vi "Renishaw-XL80_GetDX10Status.vi"(8 "error in (no error)":errorcluster, 11 "Renishaw-XL80_EMU in":refnum<class "Renishaw-XL80_EMU.lvclass">) -> (0 "error out":errorcluster, 2 "DX10Status":i32(ring) items=["DX10_CONNECTED", "DX10_NOT_RESPONDING"], 3 "Renishaw-XL80_EMU out":refnum<class "Renishaw-XL80_EMU.lvclass">)   [LabVIEW 2024, in "Renishaw-XL80_EMU.lvclass"]
doc: "DX10Status property\nThis read only property returns the current status of the DX10. It indicates whether or not the DX10 is responding.\n\nDefinition\nHRESULT\nget_DX10Status(\n [out, retval] DX10_STATUS_CODES* pVal\n);\n\nParameters\npVal\nA variable that will be set one of the DX10_STATUS_CODES.\n\nComments\nThis property will return with an HRESULT of E_FAIL if the client has not previously connected to a DX10 by calling Connect.\n\nThe property will normally return an HRESULT of S_OK. However, it will return E_POINTER if the client supplies a null pointer for pVal.\n\nNote: if there is a XL laser connected to the DX10Adaptor COM interface this property relates to a virtual DX10 and will always return DX10_CONNECTED."
uses:
  Renishaw-XL80_EMU.lvclass
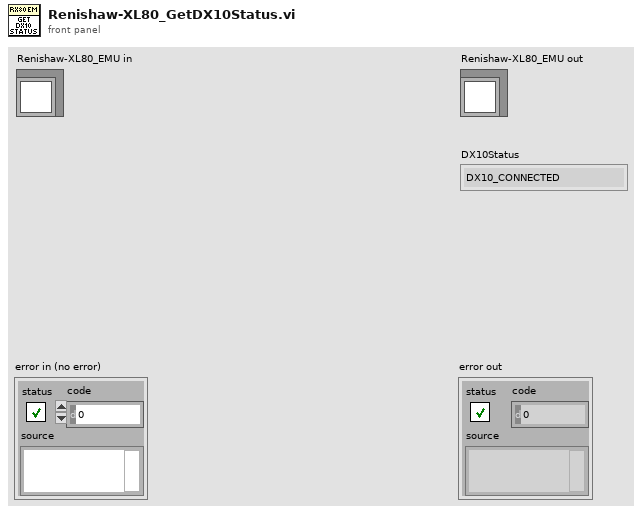
[diagram p1: front panel]
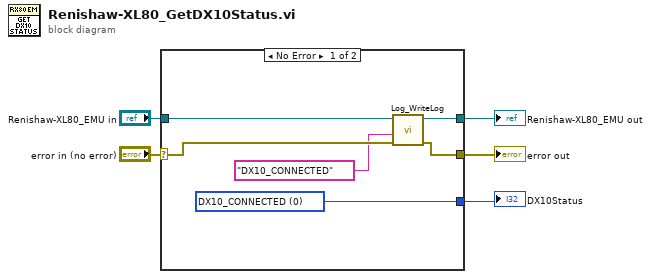
[diagram p0: block diagram]
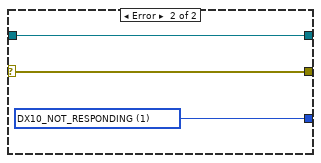
[diagram p2: hidden frame]
diagram:
  n1 = case shown="No Error" "error in (no error)" {
    selector: "error in (no error)" -> [w7 w13]
    tunnel: "Renishaw-XL80_EMU in" -> [w8 w14]
    tunnel: [w10 w14] -> w4
    tunnel: [w9 w13] -> w2
    tunnel: [w11 w12] -> w1
    frame No Error {
      w11 = 0 items=["DX10_CONNECTED", "DX10_NOT_RESPONDING"] ("DX10Status")
      n2 = call-dynamic "Log_WriteLog.vi"("error in (no error)"=w7, "Response"="DX10_CONNECTED", "Log in"=w8) -> ("error out"=w9:errorcluster, "Log out"=w10:refnum<class "Renishaw-XL80_EMU.lvclass">)  [unwired: 7 in]
    }
    frame Error {
      w12 = 1 items=["DX10_CONNECTED", "DX10_NOT_RESPONDING"] ("DX10Status")
    }
  }
  "error out" <- w2
  "Renishaw-XL80_EMU out" <- w4
  "DX10Status" <- w1
